vi "随机方块.vi"() -> (0 "方块位置信息":i32[][](array[numeric]), 2 "随机方块":bool[][](array[boolean]))   [LabVIEW 2013]
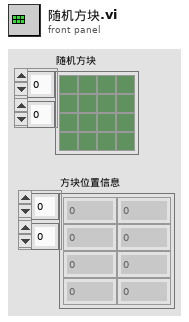
[diagram p1: front panel]
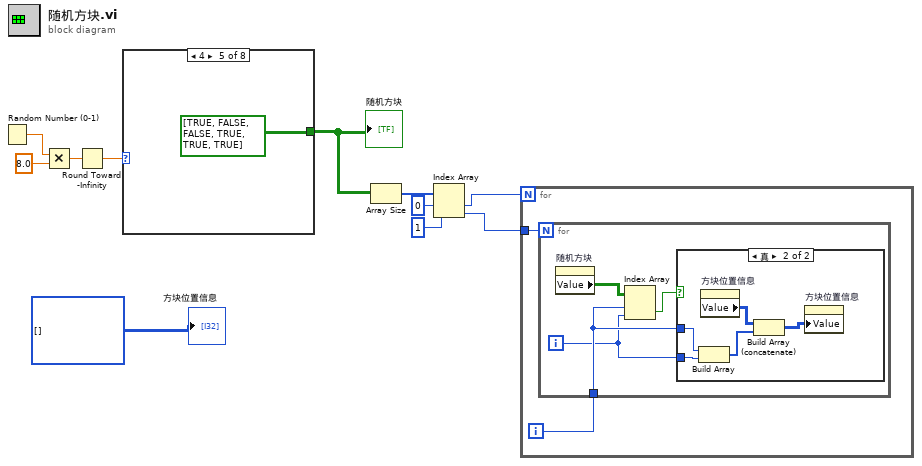
[diagram p0: block diagram]
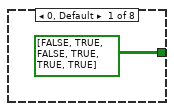
[diagram p3: hidden frame]
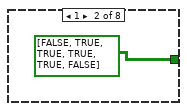
[diagram p4: hidden frame]
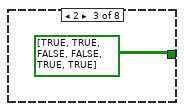
[diagram p5: hidden frame]
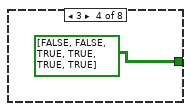
[diagram p6: hidden frame]
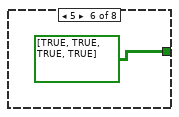
[diagram p7: hidden frame]
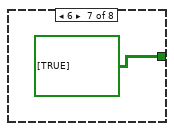
[diagram p8: hidden frame]
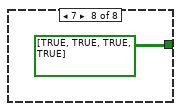
[diagram p9: hidden frame]
diagram:
  n1 = Random Number (0-1)() -> (number: 0 to 1=w10:dbl)
  n2 = Multiply(x=w10, y=8.0) -> (x*y=w9:dbl)
  n3 = Round Toward -Infinity(1:w9) -> (0:w8:dbl)
  n4 = case shown="4" w8 {
    tunnel: [bool[][] [[FALSE, TRUE, FALSE], [TRUE, TRUE, TRUE]] bool[][] [[FALSE, TRUE, TRUE], [TRUE, TRUE, FALSE]] bool[][] [[TRUE, TRUE, FALSE], [FALSE, TRUE, TRUE]] bool[][] [[FALSE, FALSE, TRUE], [TRUE, TRUE, TRUE]] bool[][] [[TRUE, FALSE, FALSE], [TRUE, TRUE, TRUE]] bool[][] [[TRUE, TRUE], [TRUE, TRUE]] bool[][] [[TRUE]] bool[][] [[TRUE, TRUE, TRUE, TRUE]]] -> w7
    frame 0, Default {
    }
    frame 1 {
    }
    frame 2 {
    }
    frame 3 {
    }
    frame 4 {
    }
    frame 5 {
    }
    frame 6 {
    }
    frame 7 {
    }
  }
  "随机方块" <- w7
  n5 = Array Size(array=w7) -> (size(s)=w6:i32[])
  n6 = Index Array(array=w6, index #1=0 ("索引"), index #2=1 ("索引")) -> (element #1=w3:i32, element #2=w2:i32)
  n7 = for {
    N: w3 -> [_]
    tunnel: w2 -> [w21]
    i -> [w20]
    n8 = for {
      N: w21 -> [_]
      tunnel: w20 -> [w23]
      i -> [w22]
      n9 = property on="随机方块" class="Arr (严格)"() -> ("Value"=w25:bool[][])  [unwired: 2 in, 2 out]
      n10 = Index Array(array=w25, index (row)=w23, index (col)=w22) -> (element=w24:bool)
      n11 = case shown="真" w24 {
        tunnel: w23 -> [_ w30]
        tunnel: w22 -> [_ w29]
        frame False {
        }
        frame True {
          n12 = Build Array(w30, w29) -> (w27:i32[])
          n13 = property on="方块位置信息" class="Arr (严格)"() -> ("Value"=w28:i32[][])  [unwired: 2 in, 2 out]
          n14 = Build Array (concatenate)(w28, w27) -> (w26:i32[][])
          n15 = property on="方块位置信息" class="Arr (严格)"("Value"=w26) -> ()  [unwired: 2 in, 2 out]
        }
      }
    }
  }
  "方块位置信息" <- i32[][] []
